vi "Get Child Information.vi"(7 "ParentID":string, 8 "error in (no error)":errorcluster, 9 "Plain Method Name in":string, 10 "Children in Memory":refnum<vi>[](array[refnum]), 11 "Queue in":refnum<queue>) -> (0 "error out":errorcluster, 3 "Queue out":refnum<queue>)   [LabVIEW 2020, in "Peek Window.lvlib" / "Dynamic Dispatch VI Type.lvclass"]
uses:
  Dynamic Dispatch VI Type.lvclass
  Implementor Tree Item Info.ctl
  Dynamic Dispatch VI Type.lvclass/Dynamic Dispatch VI Type.ctl
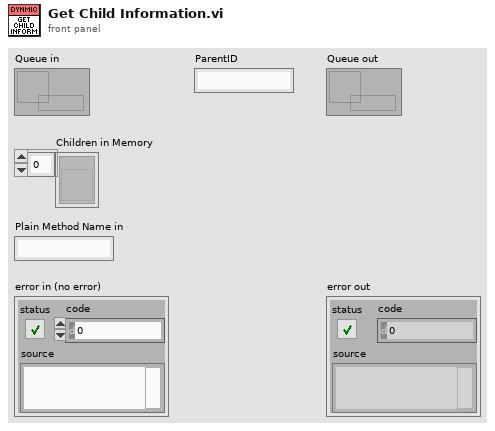
[diagram p1: front panel]
types:
  T1 = typedef "Peek Window.lvlib/Dynamic Dispatch VI Type.lvclass/Implementor Tree Item Info.ctl" = cluster{"ClassRef":refnum<vi>, "Implementor?":bool, "Parent ItemID":string, "Full Qualified Name":string}
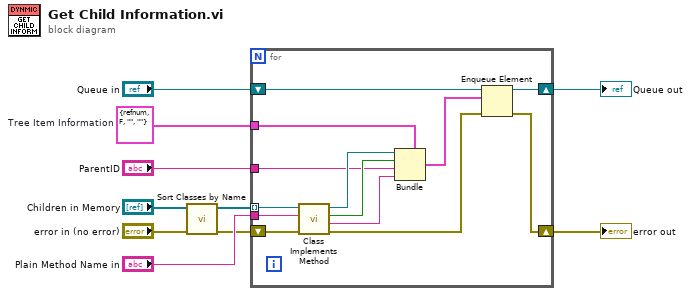
[diagram p0: block diagram]
diagram:
  w10 = T1 {"ClassRef"=refnum, "Implementor?"=FALSE, "Parent ItemID"="", "Full Qualified Name"=""}  # Tree Item Information
  n1 = call "Sort Classes by Name.vi"("error in (no error)"="error in (no error)", "Classes"="Children in Memory") -> ("error out"=w1:errorcluster, "Sorted Classes"=w3:refnum<vi>[])  [unwired: 8 in]
  n2 = for {
    tunnel: w3 -> [w19] mode=indexing
    shift-right: [w13] -> w8
    shift-left: w1 -> [w18]
    tunnel: w10 -> [w23]
    tunnel: "Plain Method Name in" -> [w17]
    shift-right: [w16] -> w7
    shift-left: "Queue in" -> [w22]
    tunnel: "ParentID" -> [w12]
    n3 = call "Class Implements Method.vi"("error in (no error)"=w18, "Method Name"=w17, "Class Refnum"=w19) -> ("error out"=w15:errorcluster, "VI Qualified Name"=w11:string, "Implements method?"=w20:bool, "Class Refnum out"=w14:refnum<vi>)  [unwired: 5 in]
    n4 = Bundle(cluster=w23, "ClassRef"=w14, "Implementor?"=w20, "Parent ItemID"=w12, "Full Qualified Name"=w11) -> (w21:T1)
    n5 = Enqueue Element(queue=w22, element=w21, error in (no error)=w15) -> (queue out=w16:refnum<queue>, error out=w13:errorcluster)  [unwired: 1 in, 1 out]
  }
  "error out" <- w8
  "Queue out" <- w7
